vi "Origin.vi"(0 "Pane in":refnum<vi>, 5 "make compliant?":bool, 7 "move all objects?":bool, 11 "error in":errorcluster) -> (4 "Pane out":refnum<vi>, 6 "non-compliant?":bool, 15 "error out":errorcluster)   [LabVIEW 2017, in "Align To Connector.lvlib"]
uses:
  Align To Connector.lvlib
  <vilib>/Utility/miscctls.llb/LVPointTypeDef.ctl
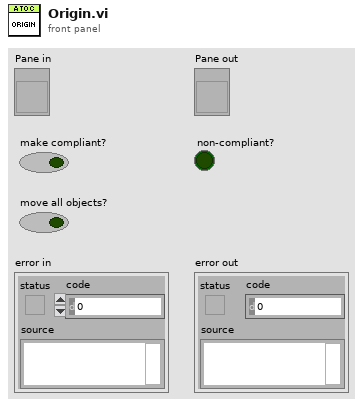
[diagram p1: front panel]
types:
  T1 = typedef "LVPointTypeDef.ctl" = cluster{"Horizontal":i16, "Vertical":i16}
  T2 = typedef "LVPositionTypeDef.ctl" = cluster{"Left":i32, "Top":i32}
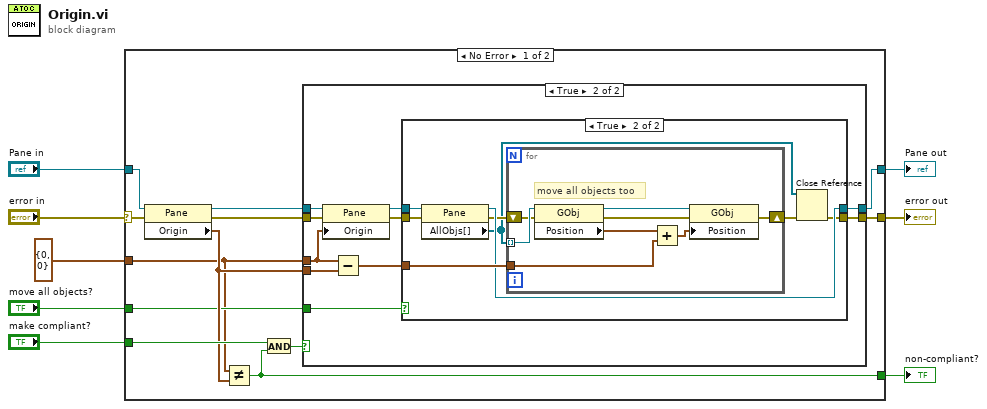
[diagram p0: block diagram]
diagram:
  n1 = case shown="No Error" "error in" {
    selector: "error in" -> [w18 w52]
    tunnel: [w10 _] -> w8
    tunnel: [w15 w52] -> w7
    tunnel: [w14 w51] -> w6
    tunnel: "Pane in" -> [w20 w51]
    tunnel: "make compliant?" -> [w19 _]
    tunnel: "move all objects?" -> [w12 _]
    tunnel: T1 {"Horizontal"=0, "Vertical"=0} ("Origin") -> [w9 _]
    frame No Error {
      n2 = property class="Pane"(reference=w20, error in=w18) -> (reference out=w16:refnum<vi>, error out=w17:errorcluster, "Origin"=w13:T1)
      n3 = Not Equal?(x=w9, y=w13) -> (x != y?=w10:bool)
      n4 = And(x=w19, y=w10) -> (x .and. y?=w11:bool)
      n5 = case shown="True" w11 {
        tunnel: w17 -> [w21 w32]
        tunnel: [w21 w27] -> w15
        tunnel: w16 -> [w22 w31]
        tunnel: [w22 w28] -> w14
        tunnel: w9 -> [_ w23]
        tunnel: w13 -> [_ w26]
        tunnel: w12 -> [_ w24]
        frame False {
        }
        frame True {
          n6 = property class="Pane"(reference=w31, error in=w32, "Origin"=w23) -> (reference out=w29:refnum<vi>, error out=w30:errorcluster)
          n7 = Subtract(x=w23, y=w26) -> (x-y=w25:T1)
          n8 = case shown="True" w24 {
            tunnel: [w33 w40] -> w28
            tunnel: w30 -> [w34 w39]
            tunnel: [w34 w36] -> w27
            tunnel: w25 -> [_ w42]
            tunnel: w29 -> [w33 w41]
            frame False {
            }
            frame True {
              n9 = property class="Pane"(reference=w41, error in=w39) -> (reference out=w40:refnum<vi>, error out=w38:errorcluster, "AllObjs[]"=w35:refnum<vi>[])
              n10 = for {
                tunnel: w35 -> [w50] mode=indexing
                shift-right: [w43] -> w37
                shift-left: w38 -> [w49]
                tunnel: w42 -> [w46]
                # "move all objects too"
                n11 = property class="GObj"(reference=w50, error in=w49) -> (reference out=w44:refnum<vi>, error out=w45:errorcluster, "Position"=w47:T2)
                n12 = Add(x=w47, y=w46) -> (x+y=w48:T2)
                n13 = property class="GObj"(reference=w44, error in=w45, "Position"=w48) -> (error out=w43:errorcluster)  [unwired: 1 out]
              }
              n14 = Close Reference(reference=w35, error in (no error)=w37) -> (error out=w36:errorcluster)
            }
          }
        }
      }
    }
    frame Error {
    }
  }
  "non-compliant?" <- w8
  "error out" <- w7
  "Pane out" <- w6
